vi "Solver.vi"(11 "Previous Guess Result":string) -> (3 "New Guess":string)   [LabVIEW 2022 SP3]
uses:
  Libraries/Wordle Engine/Wordle Engine.lvlib
panel:
  # "Note: Do not change the connector pane of this VI."
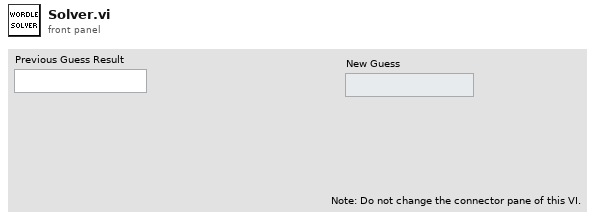
[diagram p1: front panel]
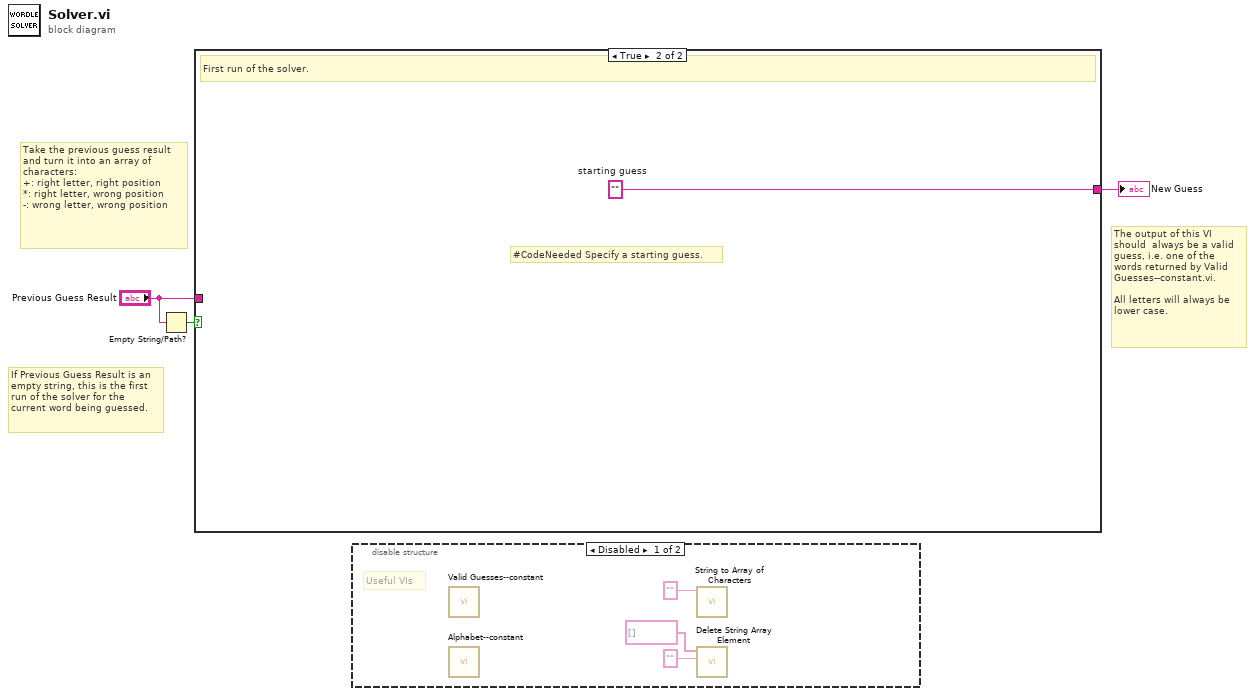
[diagram p0: block diagram]
diagram:
  # "Take the previous guess result and turn it into an array of characters:\n+: right letter, right position\n*: right letter, wrong position\n-: wrong letter, wrong position"
  # "The output of this VI should  always be a valid guess, i.e. one of the words returned by Valid Guesses--constant.vi.\n\nAll letters will always be lower case."
  # "If Previous Guess Result is an empty string, this is the first run of the solver for the current word being guessed."
  n1 = Empty String/Path?(string/path="Previous Guess Result") -> (empty?=w1:bool)
  n2 = case shown="True" w1 {
    tunnel: [_ w4] -> w3
    tunnel: "Previous Guess Result" -> [_ _]
    frame False {
      # "#CodeNeeded Add code to calculate a new guess based on the result of the previous guess. It might be good to use a Feedback Node in this VI to store data like an array of the previous guesses, which words you've eliminated from the valid guess list, etc."
      # "Non-first run of the solver."
    }
    frame True {
      w4 = ""  # starting guess
      # "#CodeNeeded Specify a starting guess."
      # "First run of the solver."
    }
  }
  "New Guess" <- w3
  n3 = disable-structure shown="Disabled" {
    frame Disabled {
      # "Useful VIs"
      n4 = call "Valid Guesses--constant.vi"() -> ()  [unwired: 10 in, 2 out]
      n5 = call "Alphabet--constant.vi"() -> ()  [unwired: 10 in, 2 out]
      n6 = call "String to Array of Characters.vi"("String"="") -> ()  [unwired: 10 in, 1 out]
      n7 = call "Delete String Array Element.vi"("Element to Delete"="", "Array in"=string[] []) -> ()  [unwired: 8 in, 2 out]
    }
    frame Enabled {
    }
  }
